vi "AlliGator Get Gate Image Series Folders.vi"(8 "Error In":errorcluster, 9 "pattern":string, 11 "Path":path) -> (0 "Error Out":errorcluster, 1 "Message":string, 2 "Timestamps":dbl[](array[numeric]), 3 "Time-Series Paths":path[](array[path]))   [LabVIEW 2021, in "AlliGator Files.lvlib"]
doc: "Reads valid folders of image in a time series."
uses:
  AlliGator Files.lvlib
  aaf9cf0a-1162-48ce-81bf-0558e63e3c5d.vi
  aaf9cf0a-1162-48ce-81bf-0558e63e3c5d.vi/f202eadf-433e-4cdb-b986-b2351ce8d73c.vi
  Strings/Strings.lvlib
  AlliGator Scripts.lvlib
  Sound/Sound.lvlib
panel:
  # "see the AlliGator License on the block diagram (Ctrl+E or Window:Show Block Diagram)"
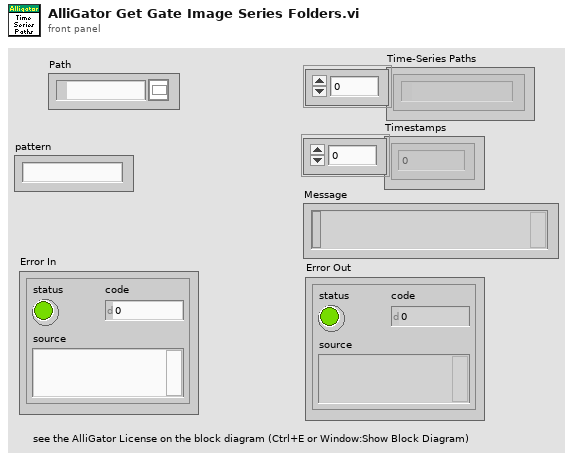
[diagram p1: front panel]
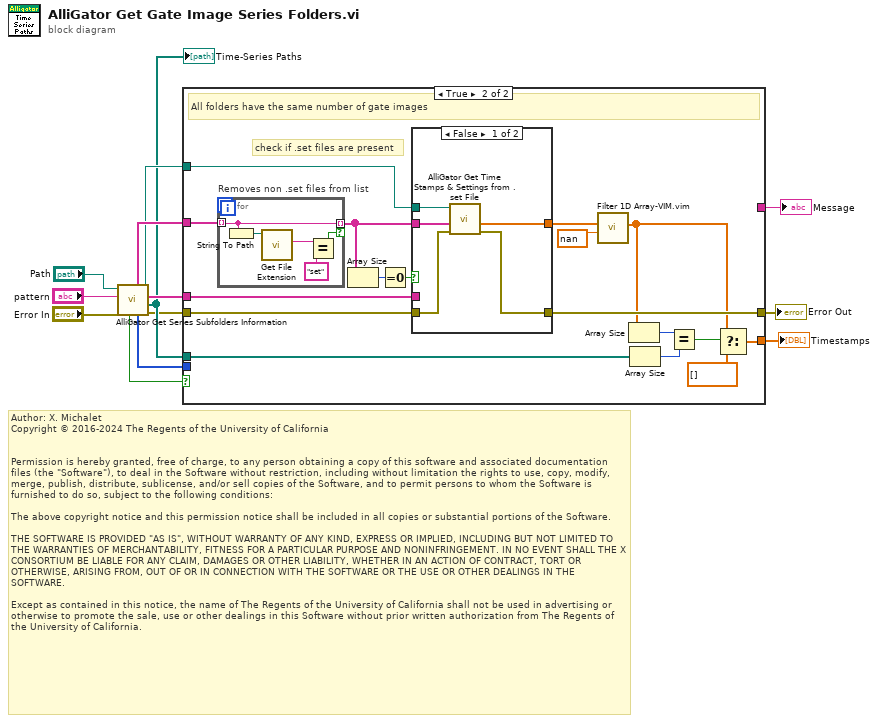
[diagram p0: block diagram]
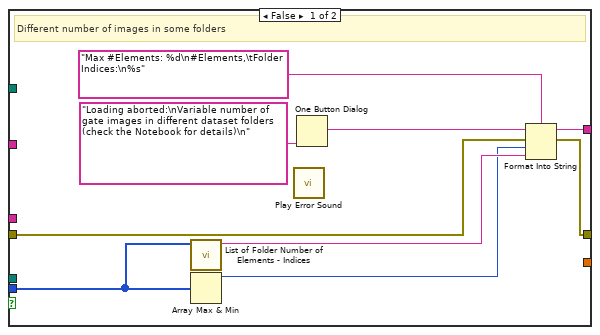
[diagram p2: hidden frame]
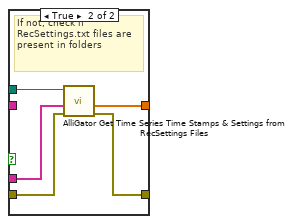
[diagram p3: hidden frame]
diagram:
  # "Author: X. Michalet\nCopyright © 2016-2024 The Regents of the University of California\n \n\nPermission is hereby granted, free of charge, to any person obtaining a copy of this software and associated documentation files (the \"Software\"), to deal in the Software without restriction, including without limitation the rights to use, copy, modify, merge, publish, distribute, sublicense, and/or sell copies of the Software, and to permit persons to whom the Software is furnished to do so, subject to the following conditions:\n\nThe above copyright notice and this permission notice shall be included in all copies or substantial portions of the Software.\n\nTHE SOFTWARE IS PROVIDED \"AS IS\", WITHOUT WARRANTY OF ANY KIND, EXPRESS OR IMPLIED, INCLUDING BUT NOT LIMITED TO THE WARRANTIES OF MERCHANTABILITY, FITNESS FOR A PARTICULAR PURPOSE AND NONINFRINGEMENT. IN NO EVENT SHALL THE X CONSORTIUM BE LIABLE FOR ANY CLAIM, DAMAGES OR OTHER LIABILITY, WHETHER IN AN ACTION OF CONTRACT, TORT OR OTHERWISE, ARISING FROM, OUT OF OR IN CONNECTION WITH THE SOFTWARE OR THE USE OR OTHER DEALINGS IN THE SOFTWARE.\n\nExcept as contained in this notice, the name of The Regents of the University of California shall not be used in advertising or otherwise to promote the sale, use or other dealings in this Software without prior written authorization from The Regents of the University of California."
  n1 = call "AlliGator Get Series Subfolders Information.vi"("error in (no error)"="Error In", "pattern"="pattern", "Path"="Path") -> ("error out"=w4:errorcluster, "Subfolder Paths"=w6:path[], "Sorted Subfolder Names"=w7:string[], "dup directory path"=w8:path, "# Files"=w1:i32[], "Files in the Root Folder"=w9:string[], "Same # Files?"=w2:bool)  [unwired: 2 in]
  "Time-Series Paths" <- w6
  n2 = case shown="True" w2 {
    tunnel: [w14 w25] -> w13
    tunnel: w8 -> [_ w27]
    tunnel: [w18 _] -> w12
    tunnel: w6 -> [_ w38]
    tunnel: [_ w34] -> w11
    tunnel: w9 -> [_ w32]
    tunnel: w4 -> [w15 w26]
    tunnel: w7 -> [_ w28]
    tunnel: w1 -> [w16 _]
    frame False {
      w21 = "Loading aborted:\nVariable number of gate images in different dataset folders (check the Notebook for details)\n" ("message")
      # "Different number of images in some folders"
      n3 = call "List of Folder Number of Elements - Indices.vi"("# Elements Array"=w16) -> ("Output String"=w19:string)  [unwired: 10 in]
      n4 = Array Max & Min(array=w16) -> (max value=w17:i32)  [unwired: 3 out]
      n5 = call "Play Error Sound.vi"() -> ()  [unwired: 27 in, 1 out]
      n6 = One Button Dialog(message=w21) -> ()  [unwired: 1 in, 1 out]
      n7 = Format Into String(format string="Max #Elements: %d\n#Elements,\tFolder Indices:\n%s", initial string=w21, error in=w15, w17, w19) -> (resulting string=w18:string, error out=w14:errorcluster)
    }
    frame True {
      # "check if .set files are present"
      # "All folders have the same number of gate images"
      n8 = for "Removes non .set files from list" {
        tunnel: w32 -> [w50] mode=indexing
        tunnel: [w50] -> w31 mode=indexing if=w49
        n9 = String To Path(string=w50) -> (path=w53:path)
        n10 = call <vilib>:"Get File Extension.vi"("file"=w53) -> ("lowercase file extension"=w52:string)  [unwired: 6 in, 4 out]
        n11 = Equal?(x=w52, y="set") -> (x = y?=w49:bool)
      }
      n12 = Array Size(array=w31) -> (size(s)=w30:i32)
      n13 = Equal To 0?(x=w30) -> (x = 0?=w29:bool)
      n14 = case shown="False" w29 {
        tunnel: w27 -> [w43 w48]
        tunnel: w31 -> [w42 _]
        tunnel: [w41 w46] -> w22
        tunnel: w28 -> [_ w47]
        tunnel: w26 -> [w40 w45]
        tunnel: [w39 w44] -> w25
        frame False {
          n15 = call "AlliGator Get Time Stamps & Settings from .set File.vi"("Error In"=w40, ".set File Names"=w42, "Folder Path"=w43) -> ("Error Out"=w39:errorcluster, "Time Stamps"=w41:dbl[])  [unwired: 6 in, 1 out]
        }
        frame True {
          # "If not, check if RecSettings.txt files are present in folders"
          n16 = call "AlliGator Get Time Series Time Stamps & Settings from RecSettings Files.vi"("Error In"=w45, "Sorted Folder Names"=w47, "Folder Path"=w48) -> ("Error Out"=w44:errorcluster, "Time Stamps"=w46:dbl[])  [unwired: 6 in, 1 out]
        }
      }
      n17 = call "Filter 1D Array-VIM.vim"("Item(s) to Filter"=nan ("Time Stamp"), "Array"=w22) -> ("Filtered Array"=w23:dbl[])  [unwired: 5 in, 1 out]
      n18 = Array Size(array=w23) -> (size(s)=w37:i32)
      n19 = Array Size(array=w38) -> (size(s)=w36:i32)
      n20 = Equal?(x=w37, y=w36) -> (x = y?=w35:bool)
      n21 = Select(t=w23, s=w35, f=dbl[] []) -> (s? t:f=w34:dbl[])
    }
  }
  "Error Out" <- w13
  "Message" <- w12
  "Timestamps" <- w11
